vi "Ignore_Allowable_Errors.vi"(8 "error in (no error)":errorcluster) -> (0 "error out":errorcluster)   [LabVIEW 2017, in "NI_ReportGenerationCore.lvlib"]
doc: "Some errors should not be propagated through the easy printing VIs. This VI will scrub the error cluster of these errors."
uses:
  <vilib>/Utility/NIReport.llb/NI_ReportGenerationCore.lvlib
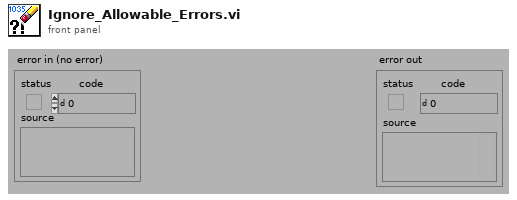
[diagram p1: front panel]
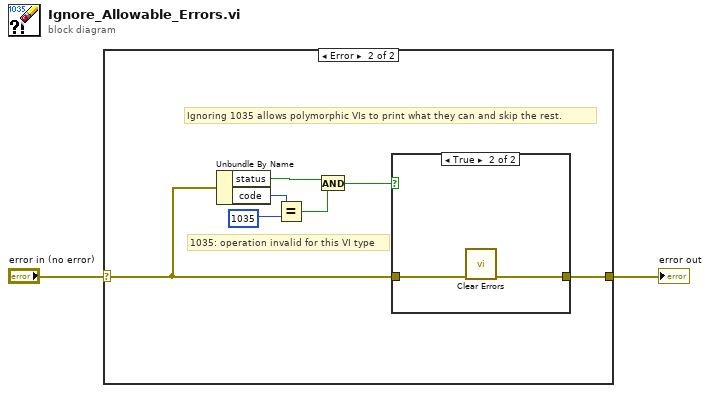
[diagram p0: block diagram]
diagram:
  n1 = case shown="Error" "error in (no error)" {
    selector: "error in (no error)" -> [w3 w5]
    tunnel: [w3 w4] -> w1
    frame No Error {
      # "To find an example VI that uses this template, select Help»Help for This VI."
    }
    frame Error {
      # "Ignoring 1035 allows polymorphic VIs to print what they can and skip the rest."
      # "1035: operation invalid for this VI type"
      n2 = Unbundle By Name(w5) -> ("status"=w8:bool, "code"=w10:i32)
      n3 = Equal?(x=w10, y=1035) -> (x = y?=w7:bool)
      n4 = And(x=w8, y=w7) -> (x .and. y?=w6:bool)
      n5 = case shown="True" w6 {
        tunnel: w5 -> [w11 w13]
        tunnel: [w11 w12] -> w4
        frame False {
        }
        frame True {
          n6 = call <vilib>:"Clear Errors.vi"("error in (no error)"=w13) -> ("error out"=w12:errorcluster)  [unwired: 5 in, 1 out]
        }
      }
    }
  }
  "error out" <- w1
